vi "Xboxinterface_86.vi"() -> (2 "R Thumb":i32(slide) scale=-32768.0..32768.0)   [LabVIEW 2009]
uses:
  <vilib>/Utility/inputDevices.llb/closeJoystick.vi
  <vilib>/Utility/inputDevices.llb/joystickAcquire.vi
panel:
  out "Log":string
  out "Start":bool
  out "Stop/Back":bool
  out "Right trigger":bool
  out "Left Trigger":bool
  out "Cluster":T1
  out "LThumb":i32(slide) scale=-32768.0..32768.0
  out "Left Thumb button":bool
  out "Right Thumb button":bool
  out "LB":bool
  out "RB":bool
  out "Y":bool
  out "X":bool
  out "B":bool
  out "A":bool caption="Boolean"
  out "joystick info":T2(array[cluster])
  out "direction info":T3
  out "button info":T4
  out "axis info":T5
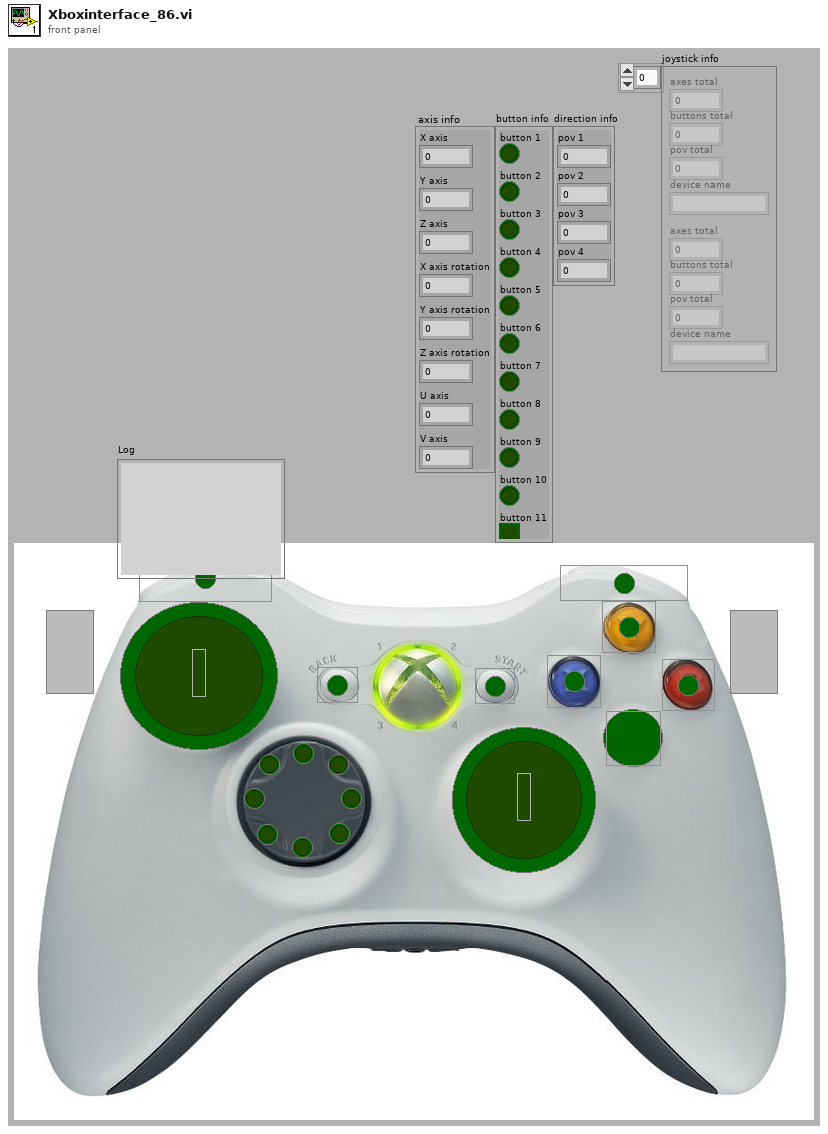
[diagram p1: front panel]
types:
  T1 = cluster{"Boolean 4":bool, "Boolean 6":bool, "Boolean 3":bool, "Boolean 7":bool, "Boolean 2":bool, "Boolean 9":bool, "Boolean 5":bool, "Boolean 8":bool}
  T2 = cluster{"axes total":u32, "buttons total":u32, "pov total":u32, "device name":string}[]
  T3 = cluster{"pov 1":i32, "pov 2":i32, "pov 3":i32, "pov 4":i32}
  T4 = cluster{"button 1":bool, "button 2":bool, "button 3":bool, "button 4":bool, "button 5":bool, "button 6":bool, "button 7":bool, "button 8":bool, "button 9":bool, "button 10":bool, "button 11":bool, "button 12":bool, "button 13":bool, "button 14":bool, "button 15":bool, "button 16":bool, "button 17":bool, "button 18":bool, "button 19":bool, "button 20":bool, "button 21":bool, "button 22":bool, "button 23":bool, "button 24":bool, "button 25":bool, "button 26":bool, "button 27":bool, "button 28":bool, "button 29":bool, "button 30":bool, "button 31":bool, "button 32":bool}
  T5 = cluster{"X axis":i32, "Y axis":i32, "Z axis":i32, "X axis rotation":i32, "Y axis rotation":i32, "Z axis rotation":i32, "U axis":i32, "V axis":i32}
  T6 = cluster{"Array[0]":bool, "Array[1]":bool, "Array[2]":bool, "Array[3]":bool, "Array[4]":bool, "Array[5]":bool, "Array[6]":bool, "Array[7]":bool}
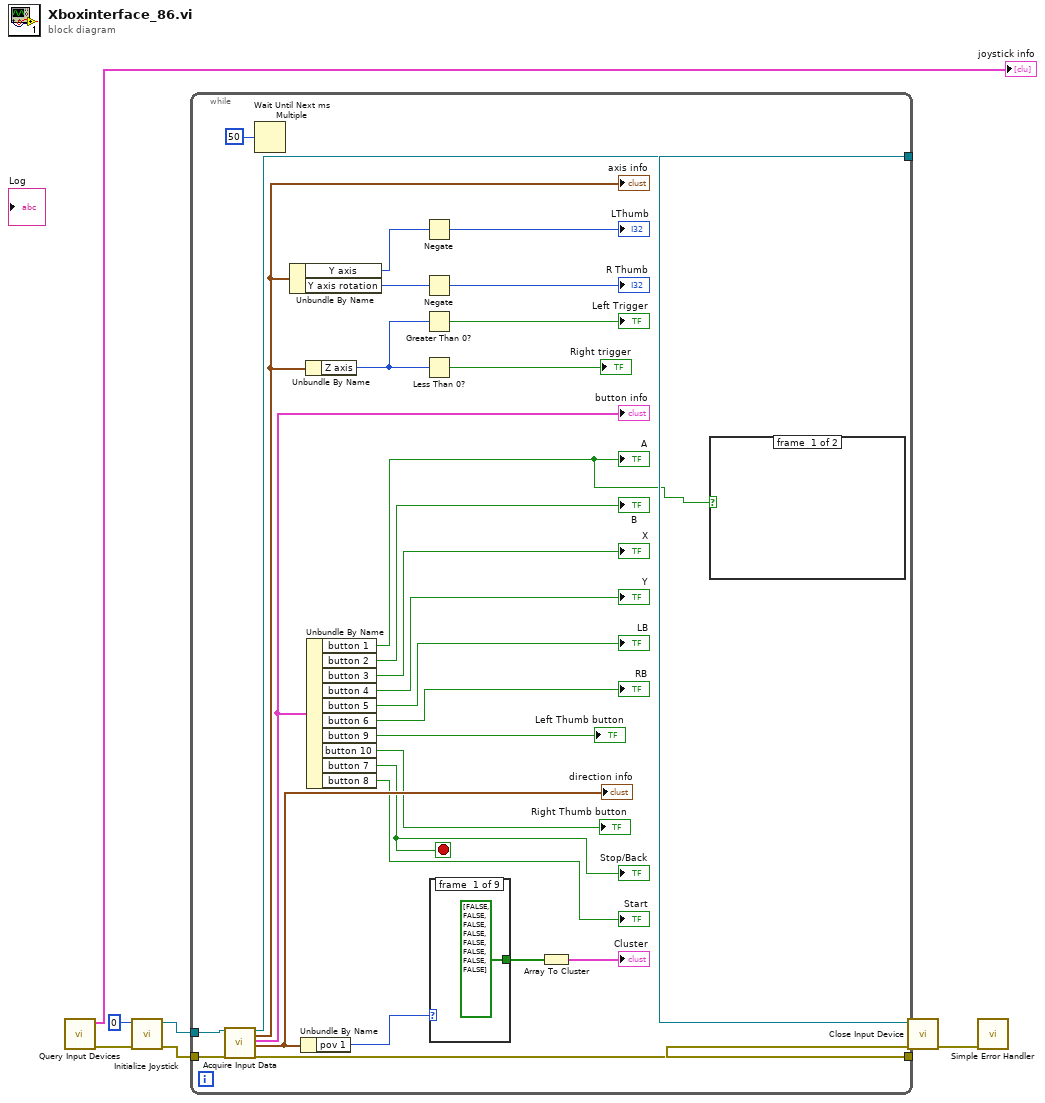
[diagram p0: block diagram]
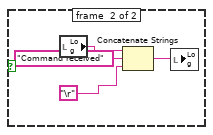
[diagram p2: hidden frame]
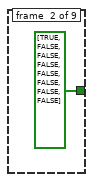
[diagram p3: hidden frame]
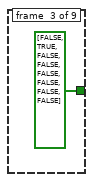
[diagram p4: hidden frame]
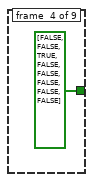
[diagram p5: hidden frame]
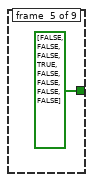
[diagram p6: hidden frame]
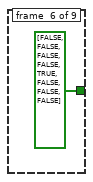
[diagram p7: hidden frame]
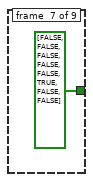
[diagram p8: hidden frame]
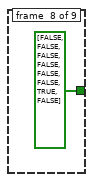
[diagram p9: hidden frame]
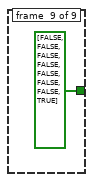
[diagram p10: hidden frame]
diagram:
  n1 = call <vilib>:"Query Input Devices.vi"() -> ("error out"=w2:errorcluster, "joystick info"=→"joystick info":T2)  [unwired: 1 in, 9 out]
  n2 = call <vilib>:"Initialize Joystick.vi"("error in (no error)"=w2, "device index"=0) -> ("error out"=w6:errorcluster, "device ID"=w7:refnum<k1>)  [unwired: 8 out]
  n3 = while {
    tunnel: w7 -> [w36]
    tunnel: w6 -> [w35]
    tunnel: [w34] -> w5
    tunnel: [w16] -> w4
    stop <- w14 stop-if-true
    n4 = call-poly <vilib>:"Acquire Input Data.vi"("device ID"=w36, "error in (no error)"=w35) -> ("device ID"=w34:refnum<k1>, "axis info"=w20:T5, "button info"=w33:T4, "direction info"=w26:T3, "error out"=w16:errorcluster)  [unwired: 13 out]
    "axis info" <- w20
    "button info" <- w33
    "direction info" <- w26
    n5 = Wait Until Next ms Multiple(millisecond multiple=u32 50) -> ()  [unwired: 1 out]
    n6 = Unbundle By Name(w20) -> ("Y axis"=w11:i32, "Y axis rotation"=w27:i32)
    n7 = Unbundle By Name(w26) -> ("pov 1"=w25:i32)
    n8 = Unbundle By Name(w20) -> ("Z axis"=w19:i32)
    n9 = Unbundle By Name(w33) -> ("button 1"=w9:bool, "button 2"=→"B":bool, "button 3"=→"X":bool, "button 4"=→"Y":bool, "button 5"=→"LB":bool, "button 6"=→"RB":bool, "button 9"=→"Left Thumb button":bool, "button 10"=→"Right Thumb button":bool, "button 7"=w14:bool, "button 8"=→"Start":bool)
    "A" <- w9
    "Stop/Back" <- w14
    n10 = Negate(x=w11) -> (-x=→"LThumb":i32)
    n11 = Negate(x=w27) -> (-x=→"R Thumb":i32)
    n12 = Greater Than 0?(x=w19) -> (x > 0?=→"Left Trigger":bool)
    n13 = Less Than 0?(x=w19) -> (x < 0?=→"Right trigger":bool)
    n14 = case shown="-1, Default" w25 {
      tunnel: [bool[] [FALSE, FALSE, FALSE, FALSE, FALSE, FALSE, FALSE, FALSE] ("Array") bool[] [TRUE, FALSE, FALSE, FALSE, FALSE, FALSE, FALSE, FALSE] ("Array") bool[] [FALSE, TRUE, FALSE, FALSE, FALSE, FALSE, FALSE, FALSE] ("Array") bool[] [FALSE, FALSE, TRUE, FALSE, FALSE, FALSE, FALSE, FALSE] ("Array") bool[] [FALSE, FALSE, FALSE, TRUE, FALSE, FALSE, FALSE, FALSE] ("Array") bool[] [FALSE, FALSE, FALSE, FALSE, TRUE, FALSE, FALSE, FALSE] ("Array") bool[] [FALSE, FALSE, FALSE, FALSE, FALSE, TRUE, FALSE, FALSE] ("Array") bool[] [FALSE, FALSE, FALSE, FALSE, FALSE, FALSE, TRUE, FALSE] ("Array") bool[] [FALSE, FALSE, FALSE, FALSE, FALSE, FALSE, FALSE, TRUE] ("Array")] -> w24
      frame #0 {
      }
      frame #1 {
      }
      frame #2 {
      }
      frame #3 {
      }
      frame #4 {
      }
      frame #5 {
      }
      frame #6 {
      }
      frame #7 {
      }
      frame #8 {
      }
    }
    n15 = Array To Cluster(array=w24) -> (cluster=→"Cluster":T6)
    n16 = case shown="True" w9 {
      frame #0 {
      }
      frame #1 {
        n17 = local read "Log"() -> (w40:string)
        n18 = Concatenate Strings(w40, "Command received" ("string"), "\r") -> (w37:string)
        n19 = local write "Log"(w37) -> ()
      }
    }
  }
  n20 = call-poly <vilib>:"Close Input Device.vi"("error in (no error)"=w4, "device ID"=w5) -> ("error out"=w1:errorcluster)  [unwired: 8 out]
  n21 = call <vilib>:"Simple Error Handler.vi"("error in (no error)"=w1) -> ()  [unwired: 1 in, 8 out]
